vi "XCL Write measurement line.vi"(6 "Iteration index":i32, 7 "report in":refnum<class "NI_report.lvclass">, 8 "error in (no error)":errorcluster, 9 "TWM result as string for XCL":string[][](array[string]), 10 "DC readings":dbl[](array[numeric]), 11 "FFmeter settings in":T1={"AC Source"={"AC Source type"=enum."Fluke 5XXX calibrator", "VISA"="", "Ref. clock (Hz)"=0.0, "status ref"=refnum}, "TWM pipe"="", "Measurement status ref"=refnum, "TWM Status ref"=refnum, "Abort ref"=refnum, "DC meter"={"DC meter type"=enum."H/A/K 3458", "DC meter VISA"="", "NPLC"=0, "status ref"=refnum}, "Measurement properties"={"Measurement frequencies (Hz)"=[], "Sampling frequency (Hz)"=0.0, "Signal amplitude (V)"=0.0, "AC-DC settle time (s)"=0.0, "Record length (multiples of period)"=[], "Measurement template file"=path "", "Row of START keyword"=0, "Row of STOP keyword"=0, "Calculate RMS from samples"=FALSE, "AC-DC warm up time (s)"=300.0, "Measurement template line"=[], "DC meter readings No."=10}, "Skip waiting ref"=refnum, "Octave paths"={"GNU Octave path"=path "C:/Program Files/GNU Octave/Octave-6.2.0/mingw64/bin", "TWM+QWTB path"=path "C:/Users/labina/Desktop/TWM-1.8.7.0-full/octprog", "lvlib path"=path "D:/martin/WAC/WACsw - github/control_software/Filter function meter/external libraries/GOLPI 0.7.3.1 source distribution LV 20.0 32 bit/lv_proc.dll"}, "Template definition"={"Keywords column"=0, "Sig. freq. column"=1, "Rec. len. column"=2, "Meas. points. row min to read"=9, "Meas. points. row max to read"=1509, "Properties column"=4, "Properties row start"=1, "Properties row end"=5, "Keyword START regexp"="", "Keyword STOP regexp"="", "HW data column"=7, "HW data row start"=1, "HW data row end"=3, "TIme and date column start"=3, "Digitizer value column start "=4, "DC mean column start "=6, "DC readings column start"=10}} {"Measurement properties"."Record length (multiples of period)" format="%#_3p"; "Measurement properties"."Sampling frequency (Hz)" format="%#_3p"; "Measurement properties"."Measurement frequencies (Hz)" format="%#_3p"}) -> (0 "error out":errorcluster, 3 "FFmeter settings out":T1={"AC Source"={"AC Source type"=enum."Fluke 5XXX calibrator", "VISA"="", "Ref. clock (Hz)"=0.0, "status ref"=refnum}, "TWM pipe"="", "Measurement status ref"=refnum, "TWM Status ref"=refnum, "Abort ref"=refnum, "DC meter"={"DC meter type"=enum."H/A/K 3458", "DC meter VISA"="", "NPLC"=0, "status ref"=refnum}, "Measurement properties"={"Measurement frequencies (Hz)"=[], "Sampling frequency (Hz)"=0.0, "Signal amplitude (V)"=0.0, "AC-DC settle time (s)"=0.0, "Record length (multiples of period)"=[], "Measurement template file"=path "", "Row of START keyword"=0, "Row of STOP keyword"=0, "Calculate RMS from samples"=FALSE, "AC-DC warm up time (s)"=300.0, "Measurement template line"=[], "DC meter readings No."=10}, "Skip waiting ref"=refnum, "Octave paths"={"GNU Octave path"=path "C:/Program Files/GNU Octave/Octave-6.2.0/mingw64/bin", "TWM+QWTB path"=path "C:/Users/labina/Desktop/TWM-1.8.7.0-full/octprog", "lvlib path"=path "D:/martin/WAC/WACsw - github/control_software/Filter function meter/external libraries/GOLPI 0.7.3.1 source distribution LV 20.0 32 bit/lv_proc.dll"}, "Template definition"={"Keywords column"=0, "Sig. freq. column"=1, "Rec. len. column"=2, "Meas. points. row min to read"=9, "Meas. points. row max to read"=1509, "Properties column"=4, "Properties row start"=1, "Properties row end"=5, "Keyword START regexp"="", "Keyword STOP regexp"="", "HW data column"=7, "HW data row start"=1, "HW data row end"=3, "TIme and date column start"=3, "Digitizer value column start "=4, "DC mean column start "=6, "DC readings column start"=10}} {"Measurement properties"."Record length (multiples of period)" format="%#_3p"; "Measurement properties"."Sampling frequency (Hz)" format="%#_3p"; "Measurement properties"."Measurement frequencies (Hz)" format="%#_3p"}, 5 "report out":refnum<class "NI_report.lvclass">)   [LabVIEW 2020]
uses:
  GUI/Type definitions/FFmeter settings.ctl
  General AC source/Type definitions/AC Source.ctl
  General AC source/Type definitions/AC Source type.ctl
  General DC meter/Type definitions/DC meter.ctl
  General DC meter/Type definitions/DC meter type.ctl
  Measurement/Type definitions/Measuement properties.ctl
  Type definitions/Template definition.ctl
  <vilib>/Utility/NIReport.llb/NI_report.lvclass
  external libraries/varilib/varilib.lvlib
  <vilib>/Analysis/NI_AALBase.lvlib
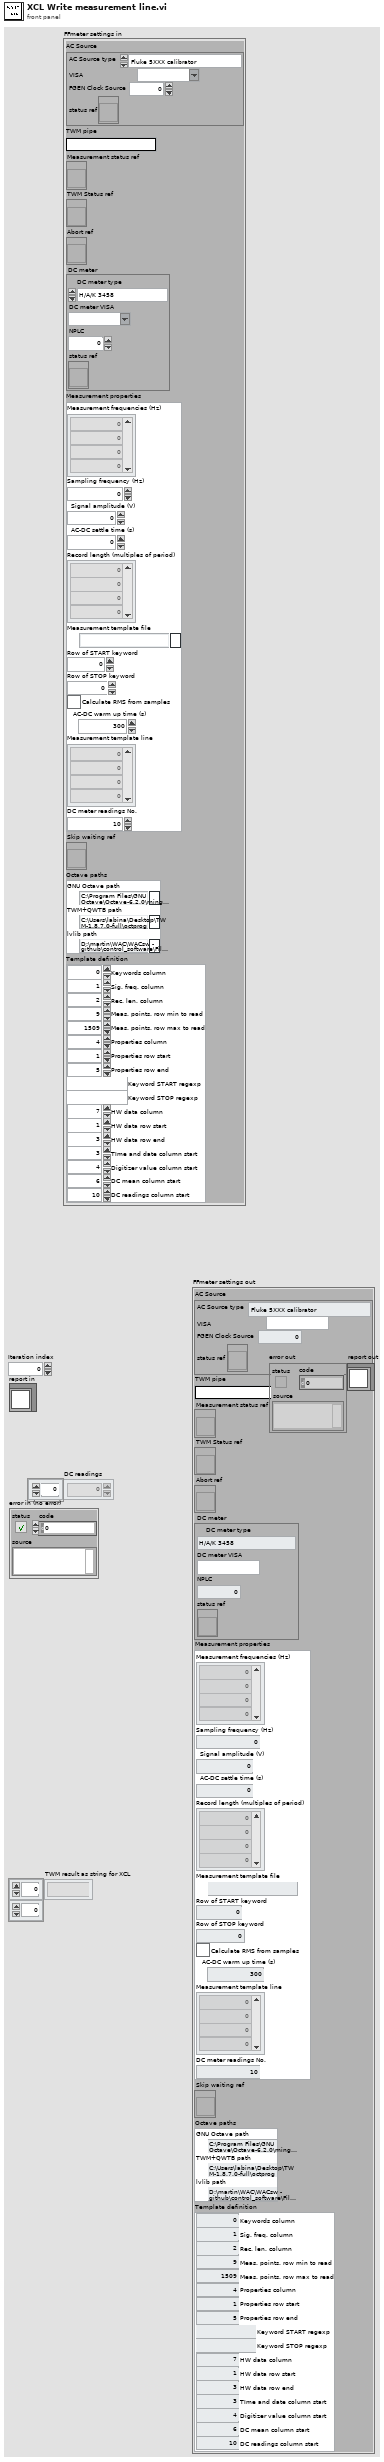
[diagram p1: front panel]
types:
  T1 = typedef "FFmeter settings.ctl" = cluster{"AC Source":T2, "TWM pipe":string, "Measurement status ref":refnum<vi>, "TWM Status ref":refnum<vi>, "Abort ref":refnum<vi>, "DC meter":T4, "Measurement properties":T6, "Skip waiting ref":refnum<vi>, "Octave paths":cluster{"GNU Octave path":path, "TWM+QWTB path":path, "lvlib path":path}, "Template definition":T7}
  T2 = typedef "AC Source.ctl" = cluster{"AC Source type":T3, "VISA":refnum<visa-resource-name>, "Ref. clock (Hz)":dbl, "status ref":refnum<vi>}
  T3 = typedef "AC Source type.ctl" = enum16{"Fluke 5XXX calibrator", "Tektronix AFG3101C", "dummy"}
  T4 = typedef "DC meter.ctl" = cluster{"DC meter type":T5, "DC meter VISA":refnum<visa-resource-name>, "NPLC":i32, "status ref":refnum<vi>}
  T5 = typedef "DC meter type.ctl" = enum16{"H/A/K 3458", "FLuke 8508A", "dummy"}
  T6 = typedef "Measuement properties.ctl" = cluster{"Measurement frequencies (Hz)":dbl[], "Sampling frequency (Hz)":dbl, "Signal amplitude (V)":dbl, "AC-DC settle time (s)":dbl, "Record length (multiples of period)":dbl[], "Measurement template file":path, "Row of START keyword":i32, "Row of STOP keyword":i32, "Calculate RMS from samples":bool, "AC-DC warm up time (s)":dbl, "Measurement template line":i32[], "DC meter readings No.":i32}
  T7 = typedef "Template definition.ctl" = cluster{"Keywords column":i32, "Sig. freq. column":i32, "Rec. len. column":i32, "Meas. points. row min to read":i32, "Meas. points. row max to read":i32, "Properties column":i32, "Properties row start":i32, "Properties row end":i32, "Keyword START regexp":string, "Keyword STOP regexp":string, "HW data column":i32, "HW data row start":i32, "HW data row end":i32, "TIme and date column start":i32, "Digitizer value column start ":i32, "DC mean column start ":i32, "DC readings column start":i32}
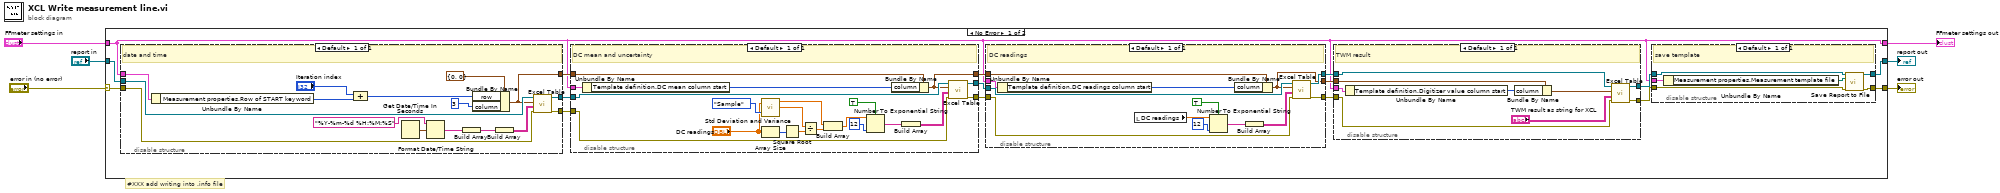
[diagram p0: block diagram]
diagram:
  # "#XXX add writing into .info file"
  n1 = case shown="No Error" "error in (no error)" {
    selector: "error in (no error)" -> [w22 w89]
    tunnel: [w20 w89] -> w6
    tunnel: "FFmeter settings in" -> [w7 w88]
    tunnel: [w7 w88] -> w3
    tunnel: "report in" -> [w21 w87]
    tunnel: [w19 w87] -> w1
    frame No Error {
      n2 = disable-structure shown="Default" {
        disable-tunnel: w22 -> [w80]
        disable-tunnel: w21 -> [w79]
        disable-tunnel: [w78] -> w18
        disable-tunnel: [w77] -> w17
        disable-tunnel: [w76] -> w16
        disable-tunnel: w7 -> [w74]
        frame Enabled {
          # "date and time"
          n3 = Unbundle By Name(w74) -> ("Measurement properties.Row of START keyword"=w73:i32)
          n4 = Compound Arithmetic op=ADD("Iteration index", w73) -> (w75:i32)
          n5 = Get Date/Time In Seconds() -> (seconds since 1Jan1904=w82:timestamp)
          n6 = Format Date/Time String(time format string (%c)="%Y-%m-%d %H:%M:%S", seconds (now)=w82) -> (date/time string=w84:string)  [unwired: 1 in]
          n7 = Build Array(w84) -> (w85:string[])
          n8 = Bundle By Name(cluster=cluster{"row":i32, "column":i32} {"row"=0, "column"=0} ("start (0, 0)"), "row"=w75, "column"=3) -> (w76:cluster{"row":i32, "column":i32})
          n9 = Build Array(w85) -> (w86:string[][])
          n10 = call "Excel Table.vi"("error in (no error)"=w80, "table"=w86, "start (0, 0)"=w76, "report in"=w79) -> ("error out"=w78:errorcluster, "report out"=w77:refnum<class "NI_report.lvclass">)  [unwired: 6 in]
        }
      }
      n11 = disable-structure shown="Default" {
        disable-tunnel: w18 -> [w68]
        disable-tunnel: w17 -> [w67]
        disable-tunnel: w16 -> [w64]
        disable-tunnel: [w63] -> w11
        disable-tunnel: [w62] -> w13
        disable-tunnel: [w61] -> w12
        disable-tunnel: w7 -> [w52]
        frame Enabled {
          # "DC mean and uncertainty"
          n12 = Unbundle By Name(w52) -> ("Template definition.DC mean column start"=w51:i32)
          n13 = call <vilib>:"Std Deviation and Variance.vi"("X"="DC readings", "Weighting (Sample)"=enum16{"Sample", "Population"}."Sample") -> ("mean"=w57:dbl, "standard deviation"=w58:dbl)  [unwired: 1 out]
          n14 = Array Size(array="DC readings") -> (size(s)=w54:i32)
          n15 = Square Root(x=w54) -> (sqrt(x)=w59:dbl)
          n16 = Divide(x=w58, y=w59) -> (x/y=w56:dbl)
          n17 = Build Array(w57, w56) -> (w55:dbl[])
          n18 = Number To Exponential String(number=w55, precision (6)=i16 12, 1:TRUE ("use system decimal point (T)")) -> (E-format string=w66:string[])  [unwired: 1 in]
          n19 = Bundle By Name(cluster=w64, "column"=w51) -> (w61:cluster{"row":i32, "column":i32})
          n20 = Build Array(w66) -> (w65:string[][])
          n21 = call "Excel Table.vi"("error in (no error)"=w68, "table"=w65, "start (0, 0)"=w61, "report in"=w67) -> ("error out"=w63:errorcluster, "report out"=w62:refnum<class "NI_report.lvclass">)  [unwired: 6 in]
        }
      }
      n22 = disable-structure shown="Default" {
        disable-tunnel: w11 -> [w39]
        disable-tunnel: w13 -> [w38]
        disable-tunnel: w12 -> [w35]
        disable-tunnel: [w34] -> w10
        disable-tunnel: [w33] -> w8
        disable-tunnel: [w32] -> w9
        disable-tunnel: w7 -> [w30]
        frame Enabled {
          # "DC readings"
          n23 = Unbundle By Name(w30) -> ("Template definition.DC readings column start"=w29:i32)
          n24 = local read "DC readings"() -> (w31:dbl[])
          n25 = Number To Exponential String(number=w31, precision (6)=i16 12, 1:TRUE ("use system decimal point (T)")) -> (E-format string=w37:string[])  [unwired: 1 in]
          n26 = Bundle By Name(cluster=w35, "column"=w29) -> (w32:cluster{"row":i32, "column":i32})
          n27 = Build Array(w37) -> (w36:string[][])
          n28 = call "Excel Table.vi"("error in (no error)"=w39, "table"=w36, "start (0, 0)"=w32, "report in"=w38) -> ("error out"=w34:errorcluster, "report out"=w33:refnum<class "NI_report.lvclass">)  [unwired: 6 in]
        }
      }
      n29 = disable-structure shown="Default" {
        disable-tunnel: w10 -> [w50]
        disable-tunnel: w8 -> [w49]
        disable-tunnel: [w48] -> w15
        disable-tunnel: [w47] -> w14
        disable-tunnel: w9 -> [w46]
        disable-tunnel: w7 -> [w43]
        frame Enabled {
          # "TWM result"
          n30 = Unbundle By Name(w43) -> ("Template definition.Digitizer value column start"=w42:i32)
          n31 = Bundle By Name(cluster=w46, "column"=w42) -> (w45:cluster{"row":i32, "column":i32})
          n32 = call "Excel Table.vi"("error in (no error)"=w50, "table"="TWM result as string for XCL", "start (0, 0)"=w45, "report in"=w49) -> ("error out"=w48:errorcluster, "report out"=w47:refnum<class "NI_report.lvclass">)  [unwired: 6 in]
        }
      }
      n33 = disable-structure shown="Default" {
        disable-tunnel: [w28] -> w20
        disable-tunnel: [w27] -> w19
        disable-tunnel: w15 -> [w26]
        disable-tunnel: w14 -> [w25]
        disable-tunnel: w7 -> [w23]
        frame Enabled {
          # "save template"
          n34 = Unbundle By Name(w23) -> ("Measurement properties.Measurement template file"=w24:path)
          n35 = call-dynamic "Save Report to File.vi"("report in"=w25, "report file path"=w24, "error in (no error)"=w26) -> ("report out"=w27:refnum<class "NI_report.lvclass">, "error out"=w28:errorcluster)  [unwired: 11 in]
        }
      }
    }
    frame Error {
    }
  }
  "FFmeter settings out" <- w3
  "error out" <- w6
  "report out" <- w1
